vi "Define macro contents with delay.vi"(0 "System no.":i32=1 min=1 max=4 step=1, 2 "Macro contents":string, 4 "milliseconds to wait":u32=5, 5 "error in":errorcluster) -> (19 "error out":errorcluster)   [LabVIEW 2020]
doc: "Defines macro contents. Each command to be stored in the macro must be written on one line, terminated with the enter key. MAC BEG.vi must be called before running this VI and MAC END.vi must be called afterwards. VI sends Macro contents one line after another separated by the specified wait time.l\n\nE-516: Macro will not be saved to FLASH until WPA .vi was run. Changes not saved with WPA are only present in RAM and will be lost when the E-516 is powered off."
panel:
  out "Array":string[](array[string])
  # "Defines macro contents. Each command to be stored in the macro must\nbe written on one line, terminated with the enter key. MAC BEG.vi must \nbe called before running this VI and MAC END.vi must be called afterwards.\nVI sends Macro contents one line after another separated by the specified\nwait time."
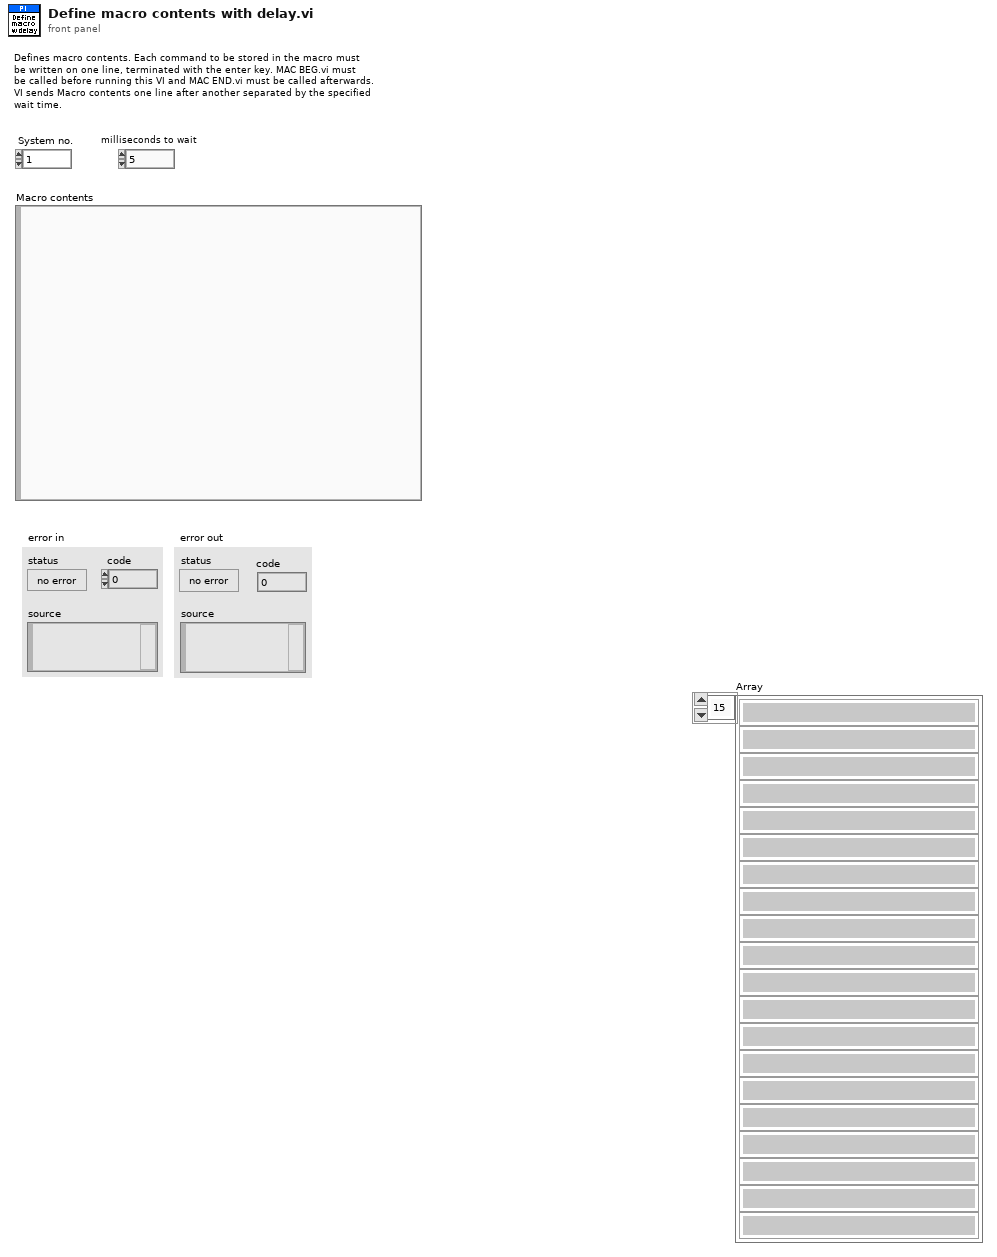
[diagram p1: front panel]
types:
  T1 = enum16{"Disable error check", "Force error check", "Use global settings"}
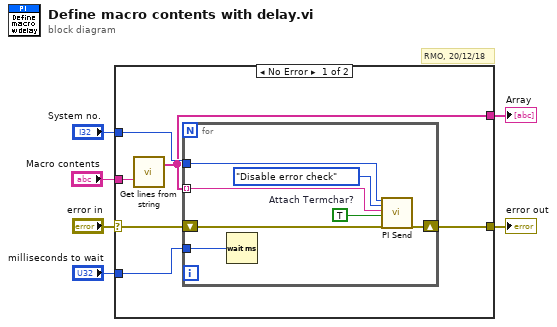
[diagram p0: block diagram]
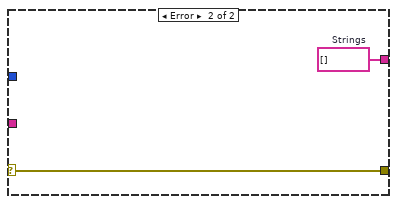
[diagram p2: hidden frame]
diagram:
  # "RMO, 20/12/18"
  n1 = case shown="No Error" "error in" {
    selector: "error in" -> [w8 w21]
    tunnel: "System no." -> [w12 _]
    tunnel: [w11 w21] -> w5
    tunnel: "milliseconds to wait" -> [w10 _]
    tunnel: "Macro contents" -> [w9 _]
    tunnel: [w7 w20] -> w1
    frame No Error {
      n2 = call "Get lines from string.vi"("Input string"=w9) -> ("Strings"=w7:string[])  [unwired: 2 in, 16 out]
      n3 = for {
        tunnel: w7 -> [w17] mode=indexing
        tunnel: w12 -> [w16]
        shift-right: [w19] -> w11
        shift-left: w8 -> [w15]
        tunnel: w10 -> [w14]
        w18 = TRUE  # Attach Termchar?
        n4 = Wait (ms)(milliseconds to wait=w14) -> ()  [unwired: 1 out]
        n5 = call "PI Send.vi"("System no."=w16, "Error check settings"=T1."Disable error check", "String to send"=w17, "Attach termination char.?"=w18, "error in"=w15) -> ("error out"=w19:errorcluster)  [unwired: 1 in, 13 out]
      }
    }
    frame Error {
      w20 = string[] []  # Strings
    }
  }
  "error out" <- w5
  "Array" <- w1
